vi "Find Calibration File.vi"(0 "Channel in":refnum<class "Channel.lvclass">, 5 "Calibration folder":path, 7 "Local folder":path, 9 "Rig":string, 11 "error in (no error)":errorcluster) -> (4 "Channel out":refnum<class "Channel.lvclass">, 6 "Calibration File":path, 15 "error out":errorcluster)   [LabVIEW 2015, in "Channel.lvclass"]
uses:
  Channel.lvclass
  Channel.lvclass/Channel.ctl
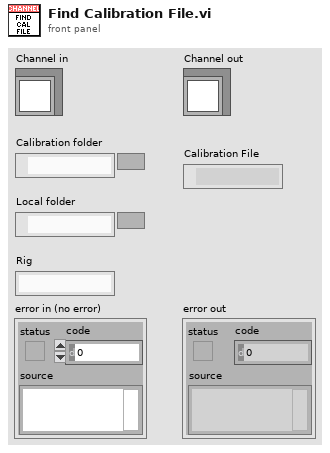
[diagram p1: front panel]
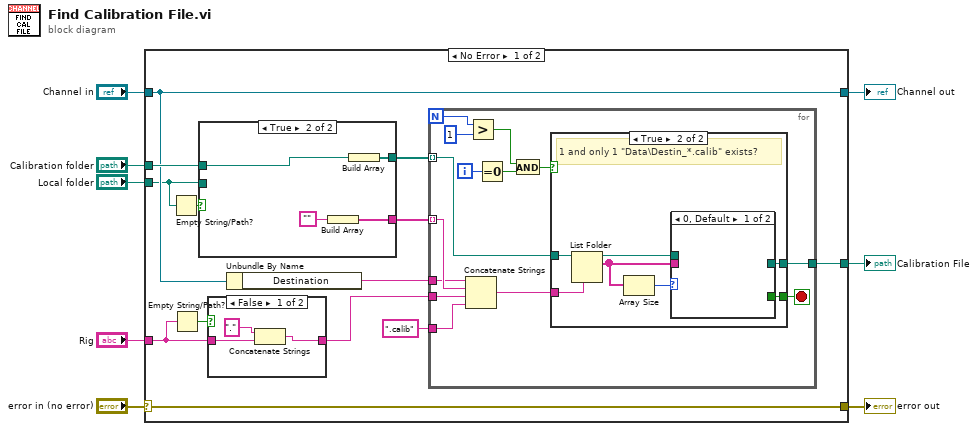
[diagram p0: block diagram]
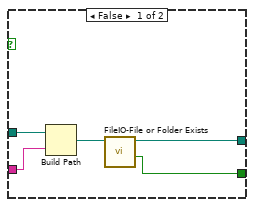
[diagram p3: hidden frame]
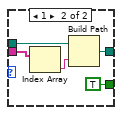
[diagram p4: hidden frame]
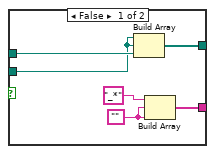
[diagram p5: hidden frame]
diagram:
  n1 = case shown="No Error" "error in (no error)" {
    selector: "error in (no error)" -> [w21 w68]
    tunnel: [w21 w68] -> w7
    tunnel: [w19 w67] -> w5
    tunnel: "Channel in" -> [w19 w67]
    tunnel: "Calibration folder" -> [w20 _]
    tunnel: "Local folder" -> [w18 _]
    tunnel: [w12 _] -> w2
    tunnel: "Rig" -> [w10 _]
    frame No Error {
      n2 = Empty String/Path?(string/path=w18) -> (empty?=w17:bool)
      n3 = Empty String/Path?(string/path=w10) -> (empty?=w11:bool)
      n4 = case shown="True" w17 {
        tunnel: w20 -> [w61 w65]
        tunnel: w18 -> [w59 _]
        tunnel: [w62 w66] -> w16
        tunnel: [w60 w64] -> w15
        frame False {
          w58 = ""
          n5 = Build Array(w59, w59, w61) -> (w62:path[])
          n6 = Build Array("_*" ("element"), w58, w58) -> (w60:string[])
        }
        frame True {
          n7 = Build Array("") -> (w64:string[])
          n8 = Build Array(w65) -> (w66:path[])
        }
      }
      n9 = case shown="False" w11 {
        tunnel: w10 -> [w24 w25]
        tunnel: [w23 w25] -> w9
        frame False {
          n10 = Concatenate Strings("." ("string"), w24) -> (w23:string)
        }
        frame True {
        }
      }
      n11 = Unbundle By Name(w19) -> ("Destination"=w14:string)
      n12 = for {
        N -> [w31]
        tunnel: w16 -> [w36] mode=indexing
        tunnel: w15 -> [w39] mode=indexing
        tunnel: w14 -> [w38]
        tunnel: ".calib" ("string") -> [w37]
        tunnel: [w34] -> w12
        tunnel: w9 -> [w32]
        i -> [w28]
        stop <- w33 stop-if-true
        n13 = Concatenate Strings(w38, w39, w32, w37) -> (w35:string)
        n14 = Greater?(x=w31, y=1) -> (0:w29:bool)
        n15 = Equal To 0?(x=w28) -> (x = 0?=w27:bool)
        n16 = And(x=w29, y=w27) -> (x .and. y?=w26:bool)
        n17 = case shown="True" w26 {
          tunnel: w36 -> [w44 w51]
          tunnel: w35 -> [w43 w50]
          tunnel: [w41 w46] -> w34
          tunnel: [w40 w45] -> w33
          frame False {
            n18 = Build Path(base path=w44, name or relative path=w43) -> (appended path=w42:path)
            n19 = call "FileIO-File or Folder Exists.vi"("path"=w42) -> ("Exists?"=w40:bool, "dup path"=w41:path)  [unwired: 7 in, 2 out]
          }
          frame True {
            # "1 and only 1 \"Data\\Destin_*.calib\" exists?"
            n20 = List Folder(path=w51, pattern=w50) -> (path out=w47:path, filenames=w48:string[])  [unwired: 2 in, 2 out]
            n21 = Array Size(array=w48) -> (size(s)=w49:i32)
            n22 = case shown="0, Default" w49 {
              tunnel: w48 -> [_ w55]
              tunnel: w47 -> [_ w56]
              tunnel: [_ w53] -> w46
              tunnel: [_ TRUE] -> w45
              frame 0, Default {
              }
              frame 1 {
                n23 = Index Array(array=w55) -> (element=w54:string)  [unwired: 1 in]
                n24 = Build Path(base path=w56, name or relative path=w54) -> (appended path=w53:path)
              }
            }
          }
        }
      }
    }
    frame Error {
    }
  }
  "error out" <- w7
  "Channel out" <- w5
  "Calibration File" <- w2
